vi "editDialog.vi"(0 "reference in":refnum<class "VINode.lvclass">, 1 "insidePackageNode":bool, 5 "error in (no error)":errorcluster) -> (14 "reference out":refnum<class "VINode.lvclass">, 15 "changeConnection":T1, 16 "cancel":bool, 19 "error out":errorcluster)   [LabVIEW 2016, in "VINode.lvclass"]
doc: "Edit Dialog"
uses:
  <resource>/Framework/Providers/Open_GDS/UML/VINode_class/VINode.lvclass
  C:/Program Files (x86)/National Instruments/LabVIEW 2016/resource/Framework/Providers/Open_GDS/UML/AbstractNode_class/AbstractNode.lvclass
  <resource>/Framework/Providers/Open_GDS/UML/AbstractNode_class/private/NodeConnectionStatsType.ctl
  <resource>/Framework/Providers/Open_GDS/UML/UMLEditor/UMLEditor_StoredPathes.ctl
  <resource>/Framework/Providers/Open_GDS/UML/ContextHelp/ContextHelp_HelpTexts.ctl
  <resource>/Framework/Providers/Open_GDS/UML/MultiLineString_class/MultiLineString.lvclass
  <resource>/Framework/Providers/Open_GDS/UML/AbstractNode_class/AbstractNode.lvclass
panel:
  in  "VIDescription":string caption="VI Description"
  in  "ShowDescription":bool caption="Show Internal Data"
  out "RelText":string="Relative path used"
  in  "Help":bool
  in  "VI Name":string
  in  "VIPath":path caption="VI Path(Optional)"
  in  "connection":bool caption="Disconnect from Package"
  in  "Cancel Button":bool
  in  "OK Button":bool
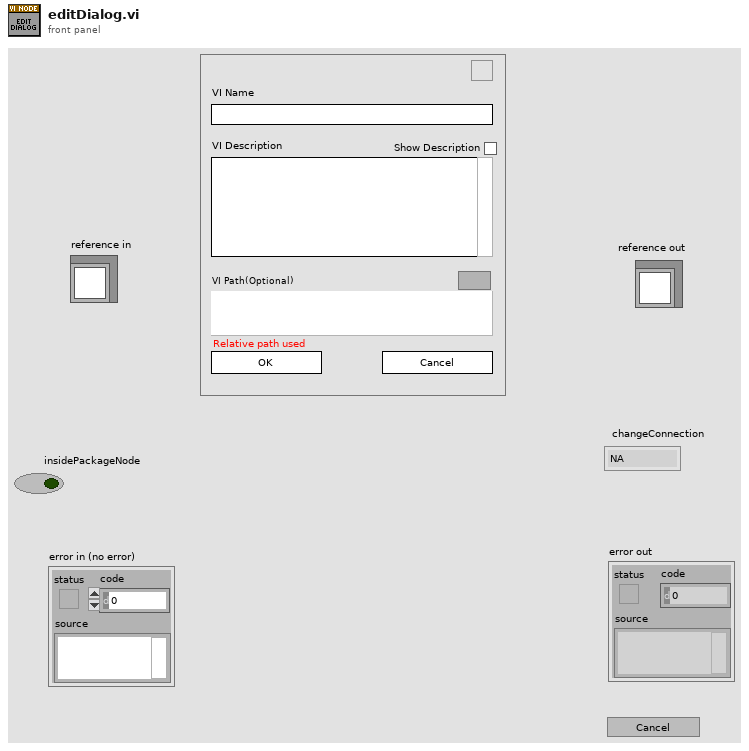
[diagram p1: front panel]
types:
  T1 = typedef "AbstractNode.lvclass/NodeConnectionStatsType.ctl" = enum16{"NA", "Connect", "DisConnect"}
  T2 = cluster{"Cancelled":bool, "Event":refnum<event-registration>, "changeConnection":T1, "Icon":u8[][]}
  T3 = typedef "UMLEditor_StoredPathes.ctl" = enum16{"LastSearchPath", "QueuedArrayStateVI", "ClassBasePath", "ViTemplatePath", "ApplicationTemplatePath", "IniFilePath", "WizDir", "RevPlugInPath"}
  T4 = cluster{"Selection Start":u32, "Selection End":u32}
  T5 = typedef "ContextHelp_HelpTexts.ctl" = enum16{"None(Hide)", "Default", "Help", "Welcome", "GettingStarted", "ClassDiagram_Help", "SequenceDiagram_Help", "UseCaseDiagram_Help", "BSelect", "BClass", "BInterface", "BPackage", "BNote", "BDependency", "BInheritance", "BInterfaceImplementation", "BAssociation", "BAggregation", "BCompAggregation", "BNoteConnector", "BObject", "BActionBar", "BCall", "BSystem", "BActor", "BUseCase", "BGeneralization", "BIncludes", "BExtends", "BUseCaseDiagramAssociation", "ClassRelationshipEdge editDialog_Bent Style", "ClassRelationshipEdge editDialog_RelationType", "ClassRelationshipEdge editDialog_Reverse association", "ClassRelationshipEdge editDialog_Start label", "ClassRelationshipEdge editDialog_Middle label", "ClassRelationshipEdge editDialog_End label", "UMLEditor reversedEngineering_Pathes", "ReversedEngineering StateReverseDialog_Help", "ReversedEngineering StateQueuedSettings_Help", "UMLEditor reversedEngineering_AddTopVIs", "UMLEditor reversedEngineering_AddClasses", "UMLEditor reversedEngineering_AddDirs", "UMLEditor reversedEngineering_Recursively", "UMLEditor reversedEngineering_Remove", "UMLEditor reversedEngineering_ClearList", "UMLEditor reversedEngineering_HideSubAss", "UMLEditor reversedEngineering_CreateTypes", "UMLEditor reversedEngineering_OnlyInheritance", "UMLEditor reversedEngineering_CreateApplication", "UMLEditor reversedEngineering_OK", "UMLEditor reversedEngineering_Cancel", "UMLEditor reversedEngineering_Help", "UMLEditor createWizardScriptFile_ScriptfilePath", "UMLEditor createWizardScriptFile_ClassPath", "UMLEditor createWizardScriptFile_Use", "UMLEditor createWizardScriptFile_PrivateDirName", "UMLEditor createWizardScriptFile_DirAppend", "UMLEditor createWizardScriptFile_Separator Character", "UMLEditor createWizardScriptFile_OK", "UMLEditor createWizardScriptFile_Cancel", "UMLEditor createWizardScriptFile_Help", "ClassNode editDialog_Class Name", "InterfaceNode editDialog_Class Name", "ClassNode editDialog_Attribute", "ClassNode editDialog_Methods", "InterfaceNode editDialog_Methods", "ClassNode editDialog_connection", "InterfaceNode editDialog_connection", "ClassNode editDialog_StereoType", "ClassNode editDialog_ShowAttrib", "ClassNode editDialog_ShowMethods", "ClassNode editDialog_ClassPath", "ClassNode editDialog_AddAttribute", "ClassNode editDialog_AddMethod", "InterfaceNode editDialog_AddMethod", "ClassNode AttributeGuide_AttributeName", "ClassNode AttributeGuide_Array?", "ClassNode AttributeGuide_Data Type", "ClassNode AttributeGuide_RefName", "ClassNode AttributeGuide_Preview", "ClassNode AttributeGuide_OK", "ClassNode AttributeGuide_Cancel", "ClassNode MethodGuide_Visibility", "ClassNode MethodGuide_Method Name", "ClassNode MethodGuide_Preview", "ClassNode MethodGuide_OK", "ClassNode MethodGuide_Cancel", "CallNode EditCallProperties_AllButtons", "ObjectNode EditObjectlProperties_AllButtons", "ActorNode EditActorProperties_AllButtons", "UseCaseRelationshipNode EditUseCaselProperties_AllButtons", "UseCaseNode EditUseCaselProperties_AllButtons", "SystemNode EditSystemProperties_AllButtons", "ReversedEngineering UpdateAttributes_AllButtons", "StateNode editDialog_AllButtons", "StateTransition editDialog_AllButtons", "ArrangeNodes Main_Picture", "ArrangeNodes Main_Zoom", "ArrangeNodes Main_Auto Zoom", "ArrangeNodes Main_shorten", "ArrangeNodes Main_Min Length", "ArrangeNodes Main_Max Length", "ArrangeNodes Main_increase", "ArrangeNodes Main_decrease", "ArrangeNodes Main_Shake", "ArrangeNodes Main", "BState", "BInitialState", "BFinalState", "BStateTransition", "StateDiagram_Help", "StateDiagram_PropertiesAllButtons", "ReversedEngineering StateReverseDialog_ClearStates", "ReversedEngineering StateReverseDialog_UseQueuedStateMachines", "ReversedEngineering StateReverseDialog_QueuedSettings", "ReversedEngineering StateReverseDialog_SearchForVIs", "ReversedEngineering StateReverseDialog_SearchCriteria", "OptionsDialog_ClassBasePath", "OptionsDialog_VIPath", "OptionsDialog_ApplicationPath", "OptionsDialog_WizDir", "OptionsDialog_IniFilePath", "OptionsDialog_DefineColors", "OptionsDialog_Help", "OptionsDialog_CreateTypes", "ClassRelationshipEdge editDialog_SplitWire"}
  T6 = typedef "VINode.lvclass/ObjectAttributes.ctl" = cluster{"midHeight":dbl, "botHeight":dbl, "Name":refnum<class "MultiLineString.lvclass">, "DEFAULT_COMPARTMENT_HEIGHT":i32, "DEFAULT_WIDTH":i32, "DEFAULT_HEIGHT":i32, "VIPath":path, "Description":refnum<class "MultiLineString.lvclass">, "ShowDescription":bool}
  T7 = typedef "AbstractNode.lvclass/ObjectAttributes.ctl" = cluster{"parent":refnum<class "AbstractNode.lvclass">, "children":refnum<class "AbstractNode.lvclass">[], "Hidden":bool}
  T8 = typedef "ContextHelp_ShowType.ctl" = cluster{"Header":string, "Picture":picture, "Text":string}
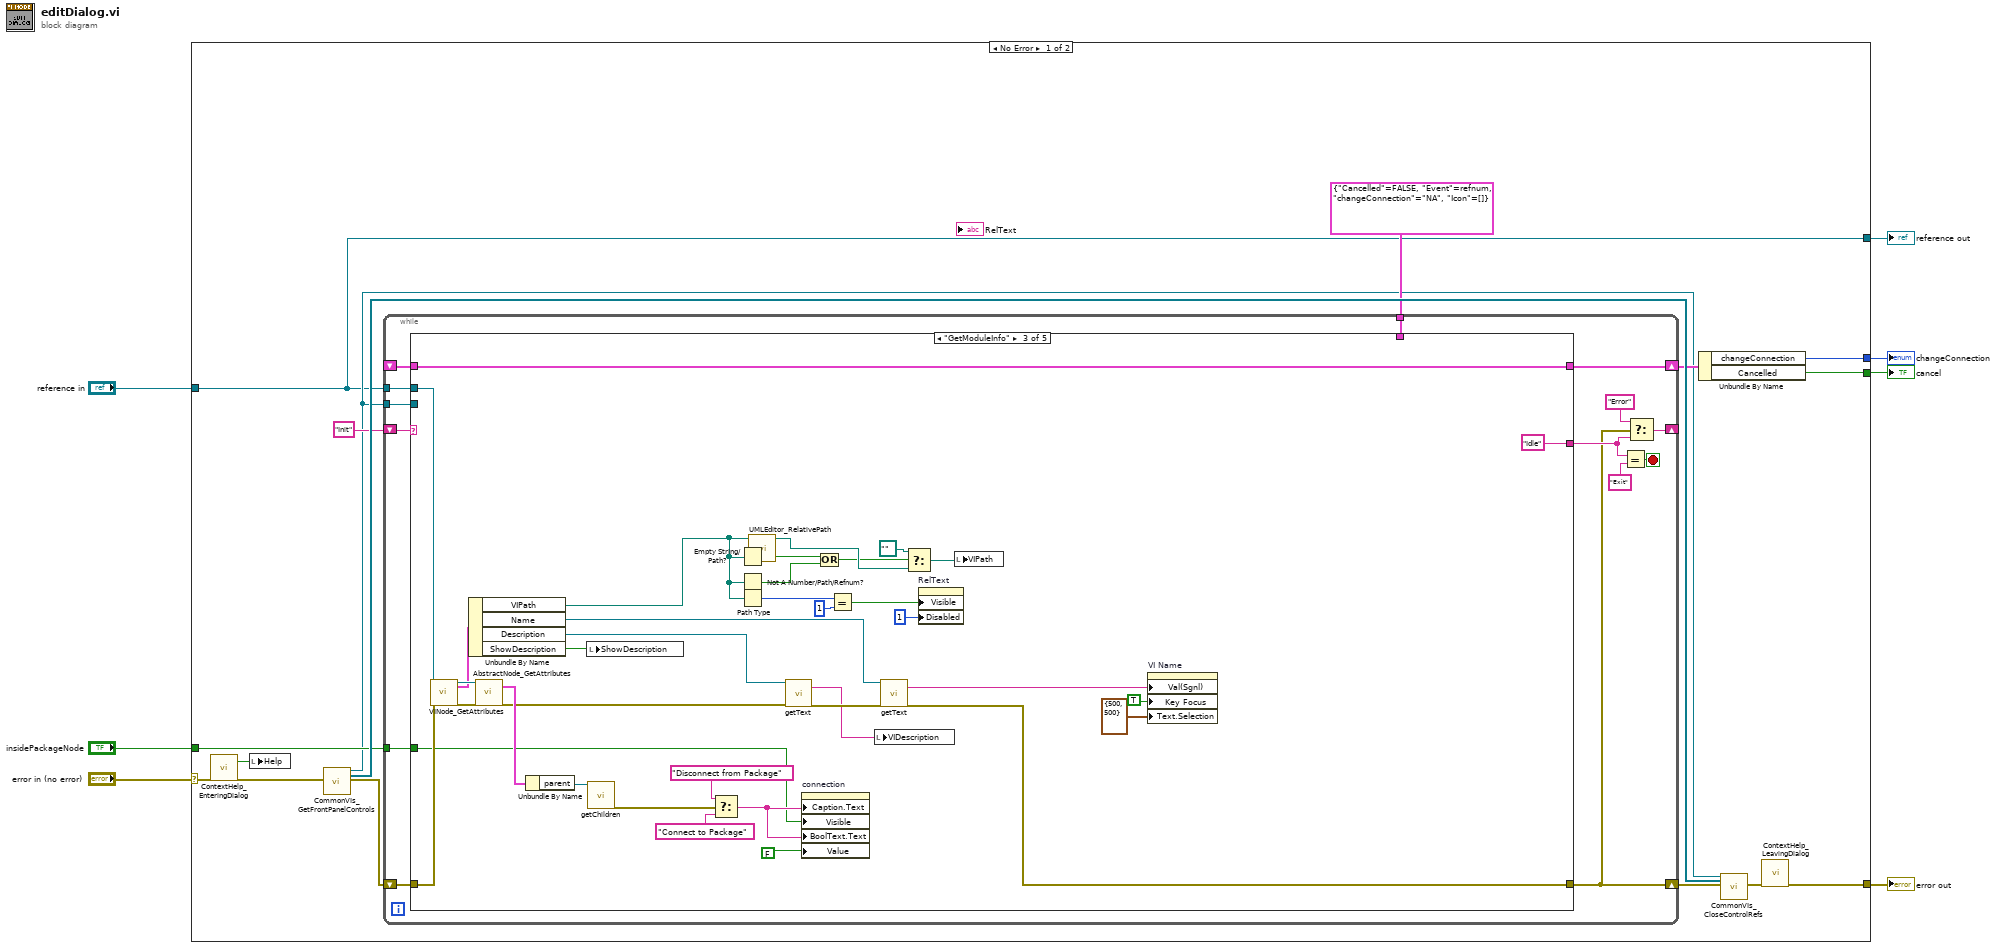
[diagram p0: block diagram]
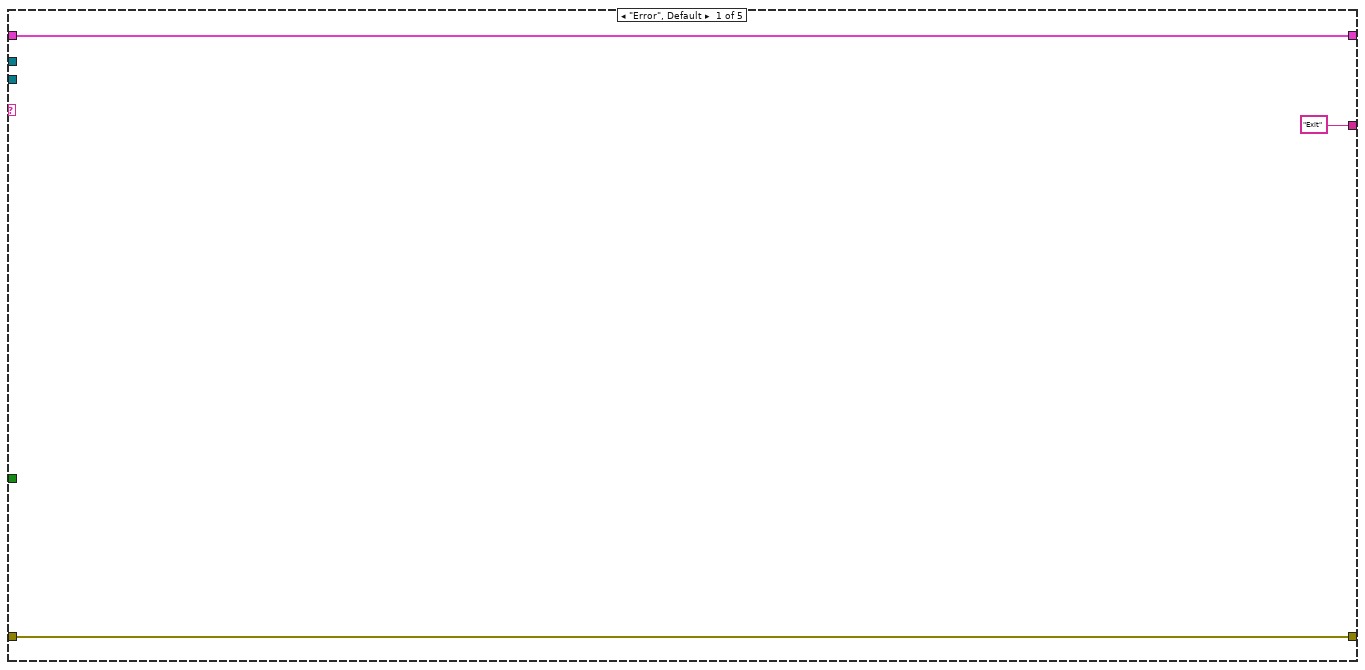
[diagram p2: hidden frame]
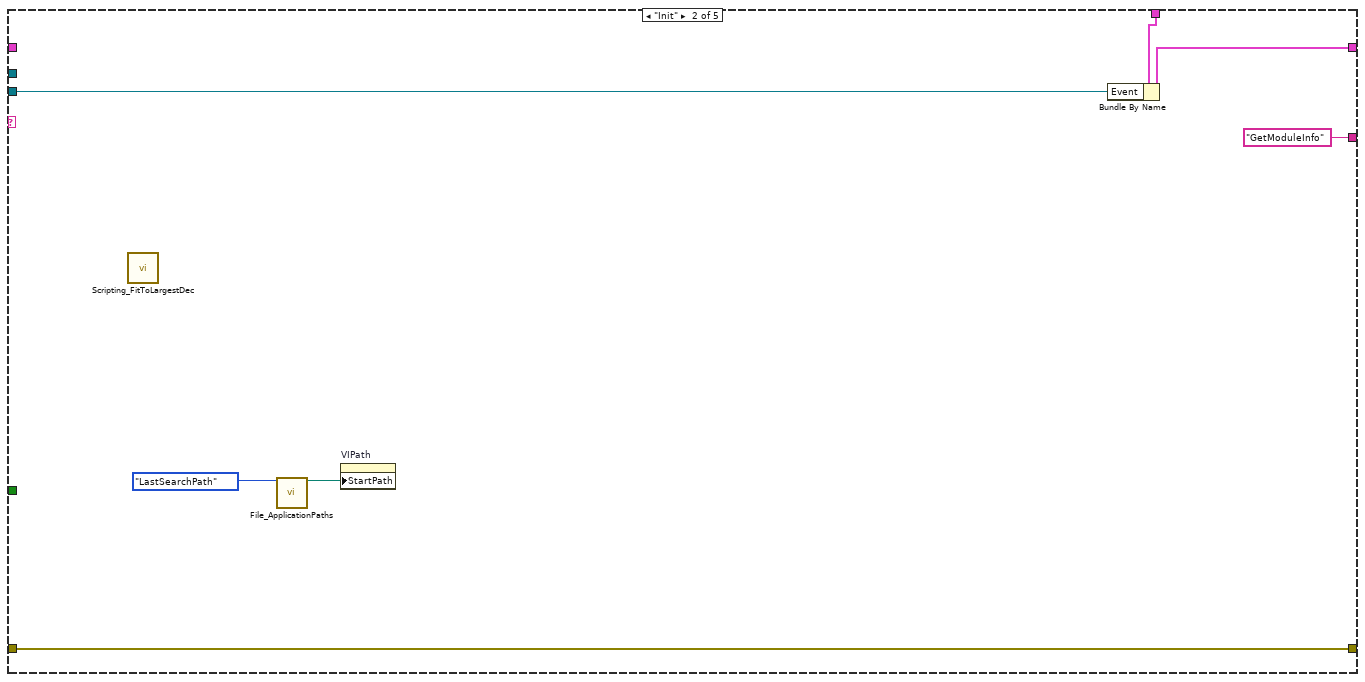
[diagram p3: hidden frame]
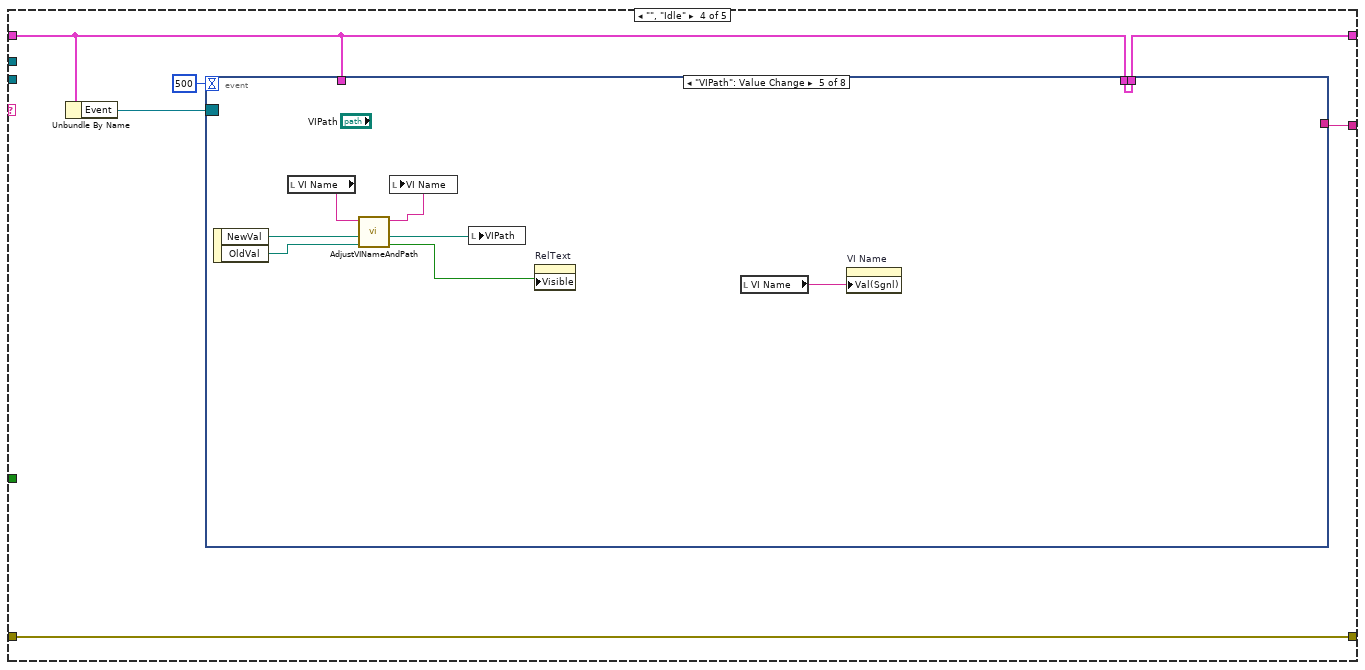
[diagram p4: hidden frame]
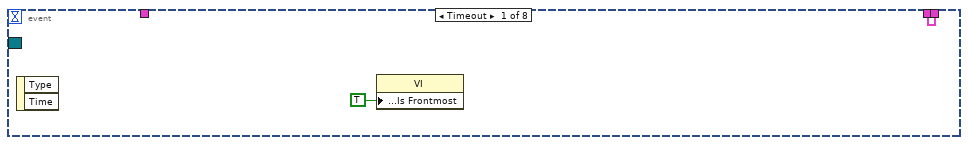
[diagram p5: hidden frame]
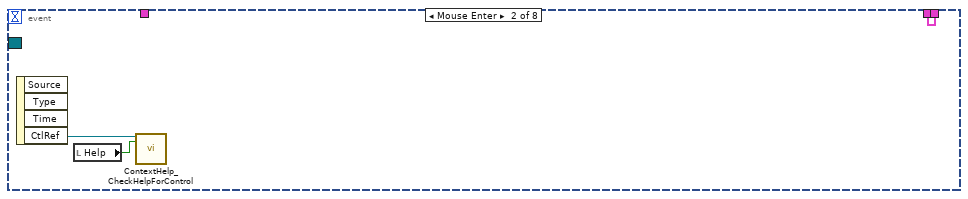
[diagram p6: hidden frame]
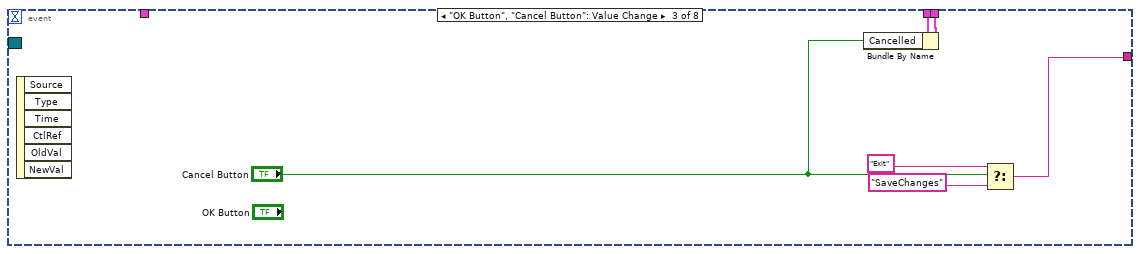
[diagram p7: hidden frame]
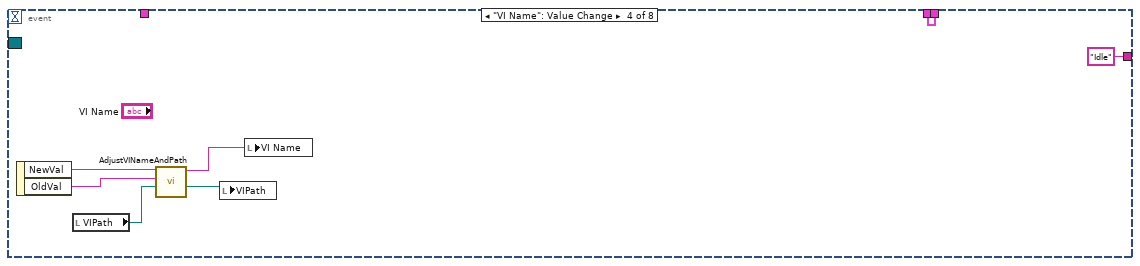
[diagram p8: hidden frame]
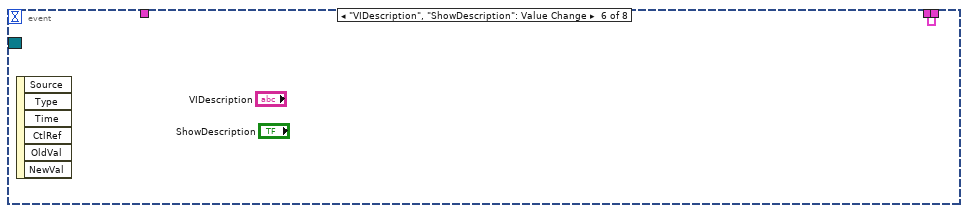
[diagram p9: hidden frame]
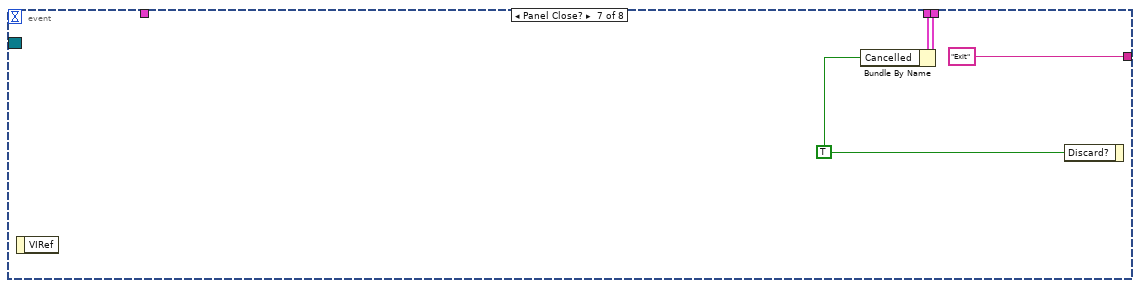
[diagram p10: hidden frame]
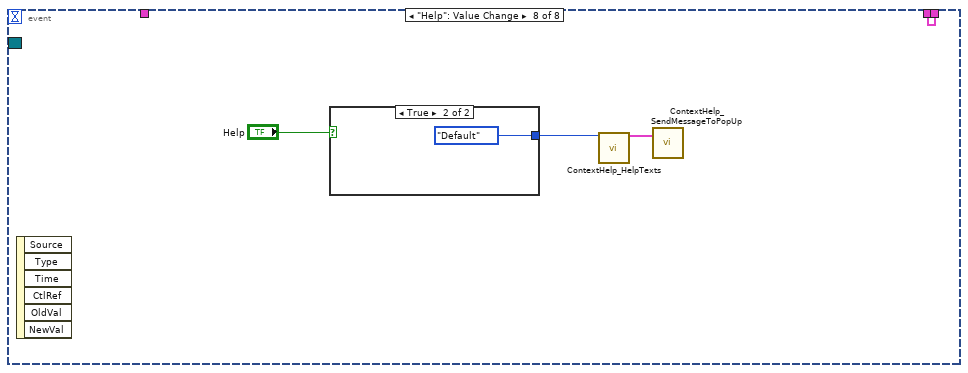
[diagram p11: hidden frame]
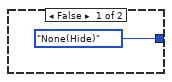
[diagram p12: hidden frame]
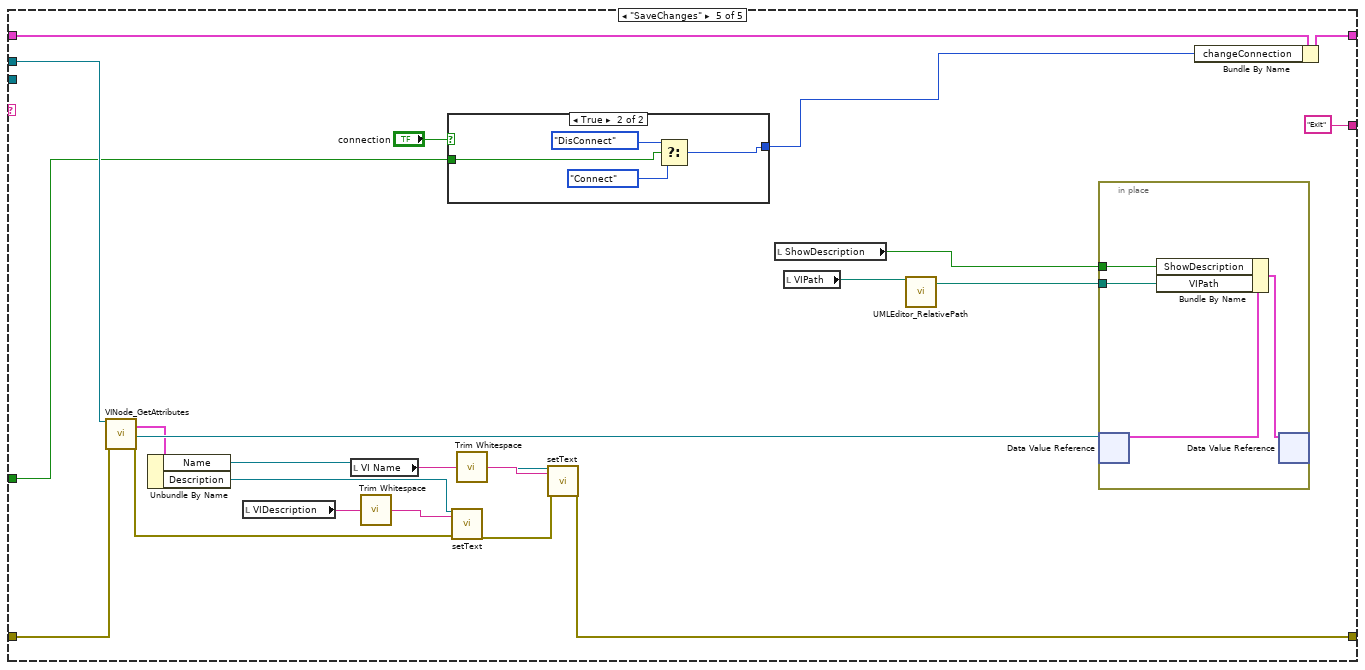
[diagram p13: hidden frame]
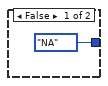
[diagram p14: hidden frame]
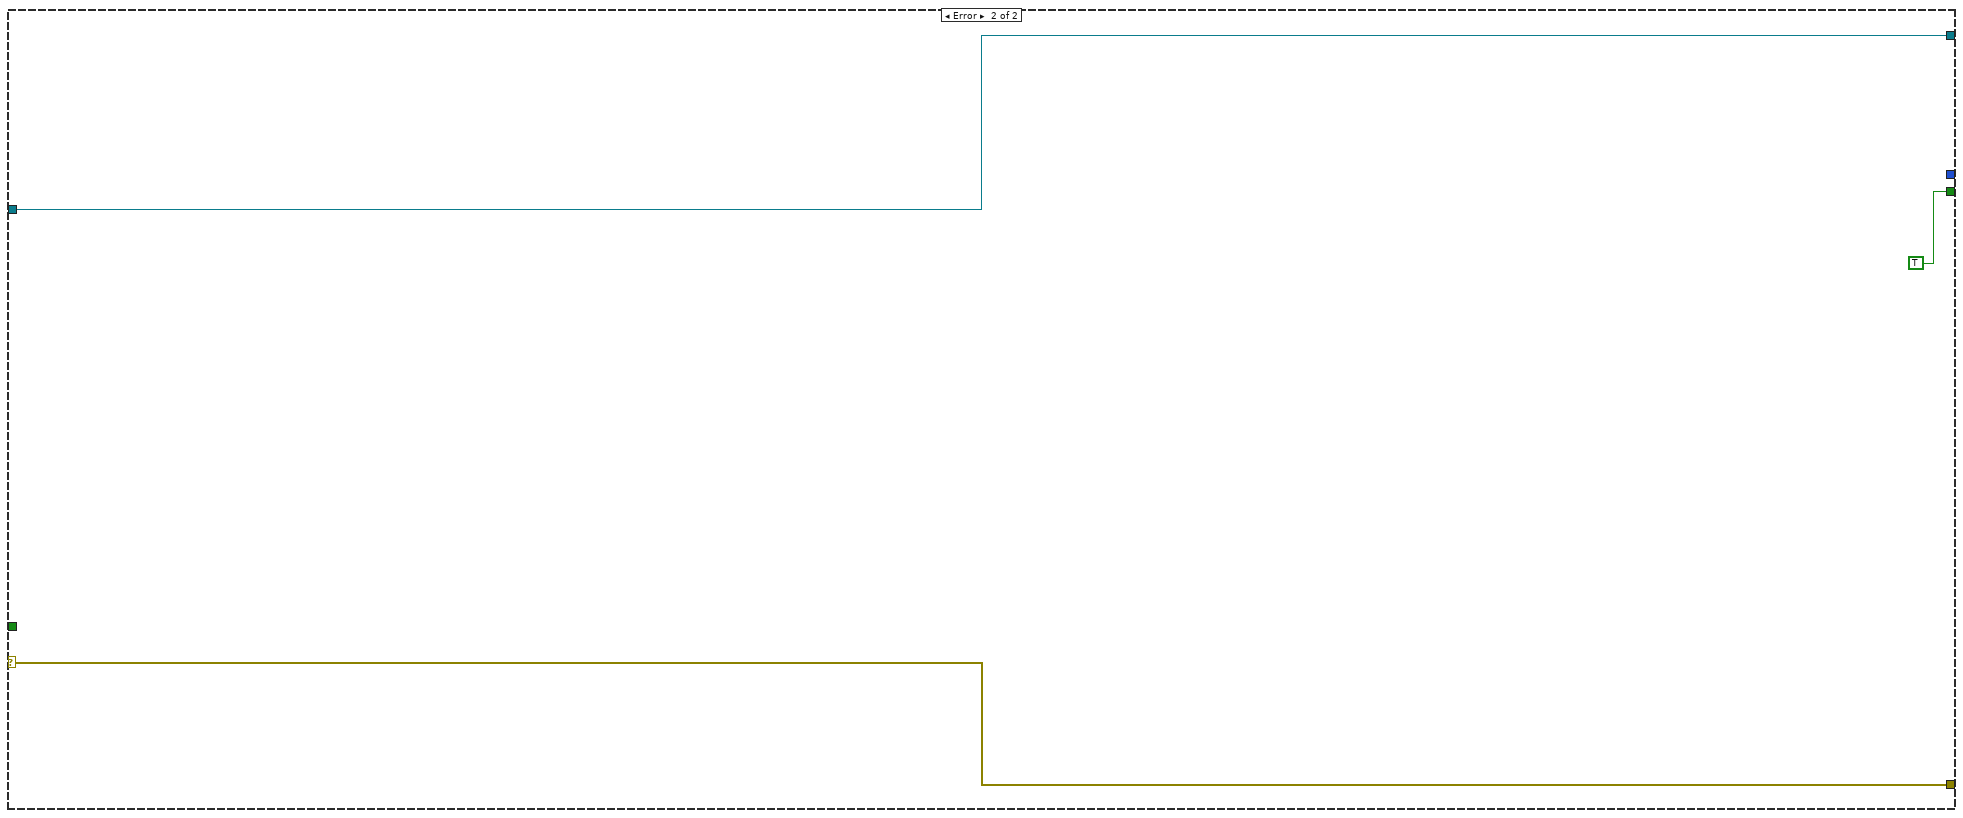
[diagram p15: hidden frame]
diagram:
  n1 = case shown="No Error" "error in (no error)" {
    selector: "error in (no error)" -> [w16 w159]
    tunnel: "reference in" -> [w8 w160]
    tunnel: [w13 w159] -> w5
    tunnel: [w8 w160] -> w4
    tunnel: "insidePackageNode" -> [w17 _]
    tunnel: [w10 _] -> w2
    tunnel: [w9 TRUE ("Key Focus")] -> w1
    frame No Error {
      n2 = call <resource>:"ContextHelp_EnteringDialog.vi"("error in (no error)"=w16) -> ("HelpStatus"=w23:bool, "error out"=w20:errorcluster)  [unwired: 2 in, 15 out]
      n3 = local write "Help"(w23) -> ()
      n4 = call <resource>:"CommonVIs_GetFrontPanelControls.vi"("error in (no error)"=w20) -> ("Event Registration Refnum"=w11:refnum<event-registration>, "ControlRefs"=w22:refnum<vi>[], "error out"=w15:errorcluster)  [unwired: 1 in, 15 out]
      n5 = while {
        shift-right: [w30] -> w14
        shift-left: w15 -> [w37]
        shift-right: [w35] -> _
        shift-left: "Init" -> [w36]
        shift-right: [w29] -> w12
        shift-left: _ -> [w28]
        tunnel: T2 {"Cancelled"=FALSE, "Event"=refnum, "changeConnection"=enum."NA", "Icon"=[]} -> [w27]
        tunnel: w17 -> [w26]
        tunnel: w11 -> [w25]
        tunnel: w8 -> [w24]
        stop <- w34 stop-if-true
        n6 = case shown="\"GetModuleInfo\"" w36 {
          tunnel: w37 -> [w40 w46 w78 w87 w138]
          tunnel: [w40 w46 w57 w87 w135] -> w30
          tunnel: ["Exit" "GetModuleInfo" "Idle" w88 "Exit"] -> w31
          tunnel: [w38 w45 w48 w89 w142] -> w29
          tunnel: w28 -> [w38 _ w48 w84 w133]
          tunnel: w27 -> [_ w44 _ _ _]
          tunnel: w26 -> [_ _ w73 _ w140]
          tunnel: w25 -> [_ w42 _ _ _]
          tunnel: w24 -> [_ _ w61 _ w143]
          frame "Error", Default {
          }
          frame "Init" {
            n7 = call <resource>:"Scripting_FitToLargestDec.vi"() -> ()  [unwired: 6 in, 2 out]
            n8 = call <resource>:"File_ApplicationPaths.vi"("PathName"=UMLEditor_StoredPathes."LastSearchPath" ("UMLPathes")) -> ("Path Out"=w43:path)  [unwired: 3 in, 15 out]
            n9 = property on="VIPath" class="Path"("StartPath"=w43) -> ()  [unwired: 2 in, 2 out]
            n10 = Bundle By Name(cluster=w44, "Event"=w42) -> (w45:T2)
          }
          frame "GetModuleInfo" {
            n11 = call <resource>:"VINode_GetAttributes.vi"("reference in"=w61, "error in (no error)"=w78) -> ("reference out"=w80:refnum<class "VINode.lvclass">, "Data"=w76:T6, "error out"=w79:errorcluster)  [unwired: 1 in, 14 out]
            n12 = Unbundle By Name(w76) -> ("VIPath"=w62:path, "Name"=w75:refnum<class "MultiLineString.lvclass">, "Description"=w50:refnum<class "MultiLineString.lvclass">, "ShowDescription"=w53:bool)
            n13 = call <resource>:"AbstractNode_GetAttributes.vi"("reference in"=w80, "error in (no error)"=w79) -> ("Data"=w77:T7, "error out"=w52:errorcluster)  [unwired: 14 in, 2 out]
            n14 = Unbundle By Name(w77) -> ("parent"=w56:refnum<class "AbstractNode.lvclass">)
            n15 = local write "ShowDescription"(w53) -> ()
            n16 = call-dynamic "getChildren.vi"("reference"=w56) -> ("error out"=w55:errorcluster)  [unwired: 15 in, 3 out]
            n17 = Select(t="Disconnect from Package", s=w55, f="Connect to Package") -> (s? t:f=w83:string)
            n18 = Empty String/Path?(string/path=w62) -> (empty?=w69:bool)
            n19 = Not A Number/Path/Refnum?(number/path/refnum=w62) -> (NaN/Path/Refnum?=w68:bool)
            n20 = Path Type(1:w62) -> (0:w64:i16)
            n21 = call <resource>:"UMLEditor_RelativePath.vi"("Path In"=w62) -> ("ConvertToAbsolutePath(If possible)"=w72:path)  [unwired: 1 in, 17 out]
            n22 = call-dynamic "getText.vi"("reference"=w50, "error in (no error)"=w52) -> ("text"=w49:string, "error out"=w51:errorcluster)  [unwired: 15 in, 1 out]
            n23 = property on="connection" class="Bool (strict)"("Caption.Text"=w83, "Visible"=w73, "BoolText.Text"=w83, "Value"=FALSE ("connection")) -> ()  [unwired: 2 in, 2 out]
            n24 = Or(x=w69, y=w68) -> (x .or. y?=w70:bool)
            n25 = Equal?(x=w64, y=i16 1) -> (x = y?=w66:bool)
            n26 = local write "VIDescription"(w49) -> ()
            n27 = call-dynamic "getText.vi"("reference"=w75, "error in (no error)"=w51) -> ("text"=w58:string, "error out"=w57:errorcluster)  [unwired: 15 in, 1 out]
            n28 = Select(t=path "", s=w70, f=w72) -> (s? t:f=w67:path)
            n29 = property on="RelText" class="Str"("Visible"=w66, "Disabled"=u8 1) -> ()  [unwired: 2 in, 2 out]
            n30 = local write "VIPath"(w67) -> ()
            n31 = property on="VI Name" class="Str"("Val(Sgnl)"=w58, "Key Focus"=TRUE, "Text.Selection"=T4 {"Selection Start"=500, "Selection End"=500}) -> ()  [unwired: 2 in, 2 out]
          }
          frame "", "Idle" {
            n32 = Unbundle By Name(w84) -> ("Event"=w86:refnum<event-registration>)
            n33 = event shown="[4] \"VIPath\": Value Change" {
              selector: w86 -> [_ _ _ _ _ _ _ _]
              dyn-events: _ -> [_ _ _ _ _ _ _ _]
              timeout: 500 -> [_ _ _ _ _ _ _ _]
              tunnel: w84 -> [w91 w94 w100 w107 w115 w116 w119 w124]
              tunnel: [w91 w94 w99 w107 w115 w116 w118 w124] -> w89
              tunnel: [_ _ w97 "Idle" _ _ "Exit" _] -> w88
              tunnel: w84 -> [_ _ _ _ _ _ _ _]
              event Timeout {
                n34 = event-data() -> ()  [unwired: 1 in, 2 out]
                n35 = property class="VI"("Front Panel Window:Is Frontmost"=TRUE) -> ()  [unwired: 2 in, 2 out]
              }
              event Mouse Enter {
                n36 = event-data() -> ("CtlRef"=w92:refnum<vi>)  [unwired: 1 in, 3 out]
                n37 = local read "Help"() -> (w93:bool)
                n38 = call <resource>:"ContextHelp_CheckHelpForControl.vi"("Ctl Refnum"=w92, "Help"=w93) -> ()  [unwired: 1 in, 17 out]
              }
              event "OK Button", "Cancel Button": Value Change {
                n39 = event-data() -> ()  [unwired: 1 in, 6 out]
                n40 = Bundle By Name(cluster=w100, "Cancelled"="Cancel Button") -> (w99:T2)
                n41 = Select(t="Exit", s="Cancel Button", f="SaveChanges") -> (s? t:f=w97:string)
              }
              event "VI Name": Value Change {
                n42 = event-data() -> ("NewVal"=w105:string, "OldVal"=w104:string)  [unwired: 1 in]
                n43 = local read "VIPath"() -> (w103:path)
                n44 = call <resource>:"AdjustVINameAndPath.vi"("NewVIPath"=w103, "OldVIName"=w104, "NewVIName"=w105) -> ("VIPath"=w102:path, "VINameOut"=w101:string)  [unwired: 6 in, 1 out]
                n45 = local write "VIPath"(w102) -> ()
                n46 = local write "VI Name"(w101) -> ()
              }
              event "VIPath": Value Change {
                n47 = event-data() -> ("NewVal"=w113:path, "OldVal"=w112:path)  [unwired: 1 in]
                n48 = local read "VI Name"() -> (w111:string)
                n49 = call <resource>:"AdjustVINameAndPath.vi"("OldVIPath"=w112, "NewVIPath"=w113, "NewVIName"=w111) -> ("RelativePath"=w108:bool, "VIPath"=w109:path, "VINameOut"=w110:string)  [unwired: 6 in]
                n50 = local write "VI Name"(w110) -> ()
                n51 = local write "VIPath"(w109) -> ()
                n52 = property on="RelText" class="Str"("Visible"=w108) -> ()  [unwired: 2 in, 2 out]
                n53 = local read "VI Name"() -> (w114:string)
                n54 = property on="VI Name" class="Str"("Val(Sgnl)"=w114) -> ()  [unwired: 2 in, 2 out]
              }
              event "VIDescription", "ShowDescription": Value Change {
                n55 = event-data() -> ()  [unwired: 1 in, 6 out]
              }
              event Panel Close? {
                w117 = TRUE ("Discard?")
                n56 = event-data() -> ()  [unwired: 1 in, 1 out]
                n57 = Bundle By Name(cluster=w119, "Cancelled"=w117) -> (w118:T2)
                n58 = event-data("Discard?"=w117) -> ()  [unwired: 1 in, 1 out]
              }
              event "Help": Value Change {
                n59 = event-data() -> ()  [unwired: 1 in, 6 out]
                n60 = case shown="True" "Help" {
                  tunnel: [ContextHelp_HelpTexts."None(Hide)" ("HelpText") ContextHelp_HelpTexts."Default" ("HelpText")] -> w122
                  frame False {
                  }
                  frame True {
                  }
                }
                n61 = call <resource>:"ContextHelp_HelpTexts.vi"("HelpText (enum or string)"=w122) -> ("HelpOut"=w121:T8)  [unwired: 18 out]
                n62 = call <resource>:"ContextHelp_SendMessageToPopUp.vi"("PopUpMessage"=w121) -> ()  [unwired: 2 in, 17 out]
              }
            }
          }
          frame "SaveChanges" {
            n63 = call <resource>:"VINode_GetAttributes.vi"("reference in"=w143, "error in (no error)"=w138) -> ("Data"=w137:T6, "DataRef"=w147:refnum<data-value>, "error out"=w131:errorcluster)  [unwired: 14 in, 1 out]
            n64 = Unbundle By Name(w137) -> ("Name"=w136:refnum<class "MultiLineString.lvclass">, "Description"=w129:refnum<class "MultiLineString.lvclass">)
            n65 = local read "VIDescription"() -> (w128:string)
            n66 = local read "VI Name"() -> (w146:string)
            n67 = call <vilib>:"Trim Whitespace.vi"("string"=w128) -> ("trimmed string"=w132:string)  [unwired: 1 in]
            n68 = case shown="True" "connection" {
              tunnel: [enum16{"NA", "Connect", "DisConnect"}."NA" ("changeConnection") w156] -> w141
              tunnel: w140 -> [_ w157]
              frame False {
              }
              frame True {
                n69 = Select(t=NodeConnectionStatsType."DisConnect" ("changeConnection"), s=w157, f=NodeConnectionStatsType."Connect" ("changeConnection")) -> (s? t:f=w156:T1)
              }
            }
            n70 = call-dynamic "setText.vi"("reference"=w129, "text"=w132, "error in (no error)"=w131) -> ("error out"=w130:errorcluster)  [unwired: 15 in, 1 out]
            n71 = call <vilib>:"Trim Whitespace.vi"("string"=w146) -> ("trimmed string"=w145:string)  [unwired: 1 in]
            n72 = call-dynamic "setText.vi"("reference"=w136, "text"=w145, "error in (no error)"=w130) -> ("error out"=w135:errorcluster)  [unwired: 15 in, 1 out]
            n73 = local read "ShowDescription"() -> (w127:bool)
            n74 = local read "VIPath"() -> (w134:path)
            n75 = call <resource>:"UMLEditor_RelativePath.vi"("Path In"=w134) -> ("ConvertToRelativePath(If possible)"=w148:path)  [unwired: 1 in, 17 out]
            n76 = in-place {
              in-place-border: w148 -> [w150]
              in-place-border: w127 -> [w149]
              n77 = in-place-dvr #1(w147) -> (w152:T6)  [unwired: 1 out]
              n78 = Bundle By Name(cluster=w152, "ShowDescription"=w149, "VIPath"=w150) -> (w151:T6)
              n79 = in-place-dvr #1(w151) -> ()  [unwired: 2 out]
            }
            n80 = Bundle By Name(cluster=w133, "changeConnection"=w141) -> (w142:T2)
          }
        }
        n81 = Equal?(x=w31, y="Exit") -> (x = y?=w34:bool)
        n82 = Select(t="Error", s=w30, f=w31) -> (s? t:f=w35:string)
      }
      n83 = Unbundle By Name(w12) -> ("changeConnection"=w10:T1, "Cancelled"=w9:bool)
      n84 = call <resource>:"CommonVIs_CloseControlRefs.vi"("Event Registration Refnum"=w11, "ControlRefs"=w22, "error in (no error)"=w14) -> ("error out"=w21:errorcluster)  [unwired: 16 out]
      n85 = call <resource>:"ContextHelp_LeavingDialog.vi"("error in (no error)"=w21) -> ("error out"=w13:errorcluster)  [unwired: 2 in, 16 out]
    }
    frame Error {
    }
  }
  "reference out" <- w4
  "error out" <- w5
  "changeConnection" <- w2
  "cancel" <- w1
